vi "Pulse thingy.vi"() -> ()   [LabVIEW 2015]
uses:
  <vilib>/express/express analysis/Spectral/Block/exnSpectralBlock spectral measurements RMS poly.vi
  <vilib>/express/express analysis/Spectral/Block/exnSpectralBlock spectral measurements RMS WFM.vi
  <vilib>/express/express analysis/Spectral/XNode/ExpressSpectralMeasurementsBlockNode.xnode
panel:
  out "Time Graph":waveform(dbl)(graph)
  out "FFT Graph":cluster{"f0":dbl, "df":dbl, "magnitude":dbl[]}(graph)
  in  "Time":dbl
  in  "Rate":dbl
  in  "Averages":dbl
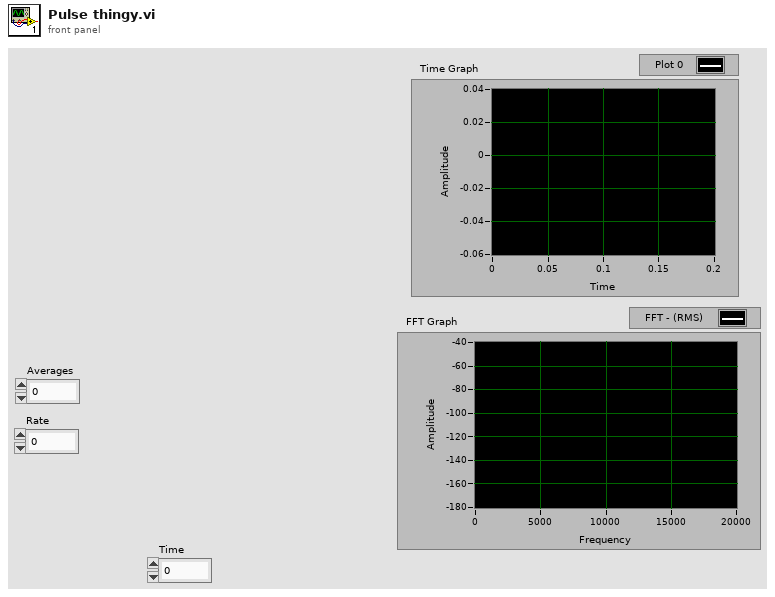
[diagram p1: front panel]
types:
  T1 = cluster{"averaging mode":u16, "weighting mode":u16, "number of averages":u32}
  T2 = cluster{"dB On (F)":bool, "unwrap phase (F)":bool, "convert to degree (F)":bool}
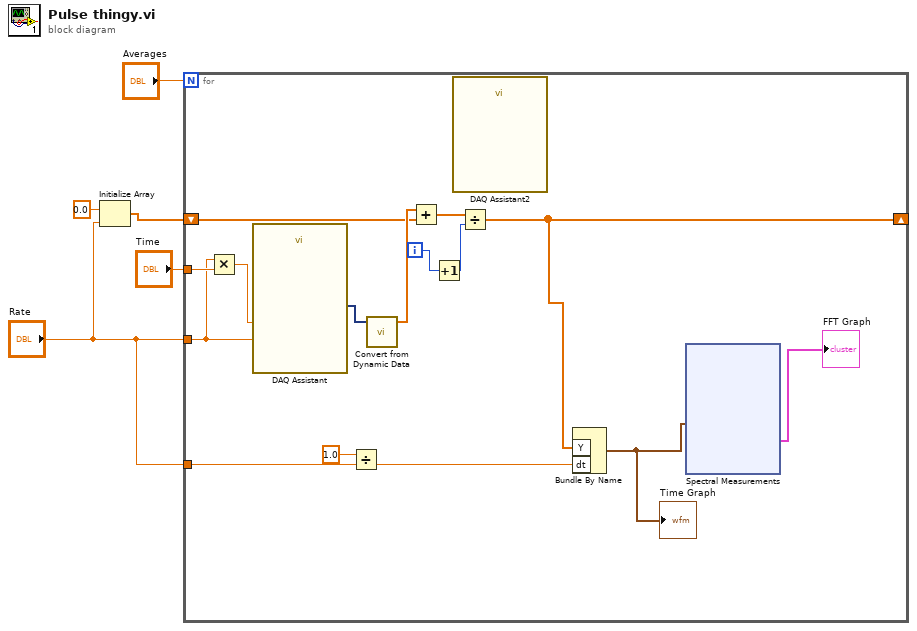
[diagram p0: block diagram]
diagram:
  n1 = Initialize Array(0.0 ("element"), "Rate") -> (w3:dbl[])
  n2 = for {
    N: "Averages" -> [_]
    tunnel: "Rate" -> [w19]
    tunnel: "Time" -> [w20]
    shift-right: [w8] -> _
    shift-left: w3 -> [w15]
    tunnel: "Rate" -> [w11]
    i -> [w17]
    n3 = Multiply(x=w19, y=w20) -> (x*y=w18:dbl)
    n4 = call "DAQ Assistant"("rate"=w19, "number of samples"=w18) -> ("data"=w12:dynamicdata)  [unwired: 15 in, 2 out]
    n5 = Divide(x=1.0, y=w11) -> (x/y=w10:dbl)
    n6 = call "Convert from Dynamic Data"("Dynamic Data Type"=w12) -> ("Array"=w16:dbl[])  [unwired: 3 in]
    n7 = Add(x=w16, y=w15) -> (x+y=w14:dbl[])
    n8 = Increment(x=w17) -> (x+1=w13:i32)
    n9 = call "DAQ Assistant2"() -> ()  [unwired: 18 in, 2 out]
    n10 = Divide(x=w14, y=w13) -> (x/y=w8:dbl[])
    n11 = Bundle By Name("Y"=w8, "dt"=w10) -> (w7:waveform(dbl))  [unwired: 1 in]
    "Time Graph" <- w7
    n12 = xnode "Spectral Measurements"("Signals"=w7) -> ("FFT - (RMS)"=→"FFT Graph":cluster{"f0":dbl, "df":dbl, "magnitude":dbl[]})  [unwired: 1 in, 2 out]
  }
